vi "Read Resource Name.vi"(8 "error in (no error)":errorcluster, 11 "Abstract Switch Init Parameters in":refnum<class "Abstract Switch Init Parameters.lvclass">) -> (0 "error out":errorcluster, 2 "Resource Name":string, 3 "Abstract Switch Init Parameters out":refnum<class "Abstract Switch Init Parameters.lvclass">)   [LabVIEW 2017, in "Messaging.lvlib" / "Abstract Switch Init Parameters.lvclass"]
uses:
  Abstract Switch Init Parameters.lvclass
  Abstract Switch Init Parameters.lvclass/Abstract Switch Init Parameters.ctl
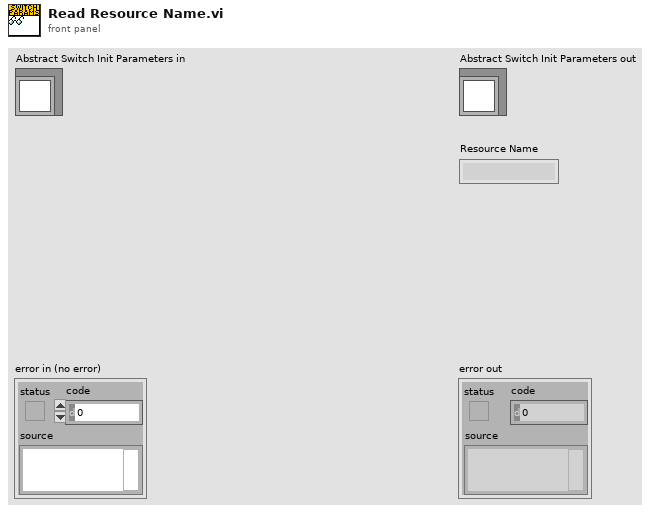
[diagram p1: front panel]
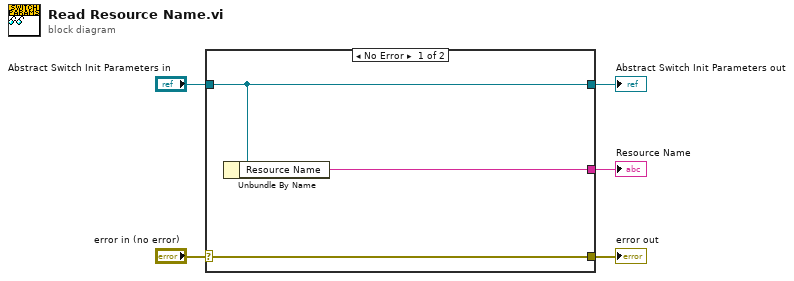
[diagram p0: block diagram]
diagram:
  n1 = case shown="No Error" "error in (no error)" {
    selector: "error in (no error)" -> [w8 w9]
    tunnel: [w8 w9] -> w4
    tunnel: [w7 w10] -> w2
    tunnel: "Abstract Switch Init Parameters in" -> [w7 w10]
    tunnel: [w6 _] -> w1
    frame No Error {
      n2 = Unbundle By Name(w7) -> ("Resource Name"=w6:string)
    }
    frame Error {
    }
  }
  "error out" <- w4
  "Abstract Switch Init Parameters out" <- w2
  "Resource Name" <- w1
